vi "sigmoid.vi"(11 "x":dbl) -> (3 "sigmoid(x)":dbl)   [LabVIEW 2019]
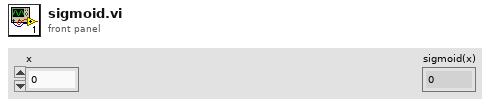
[diagram p1: front panel]
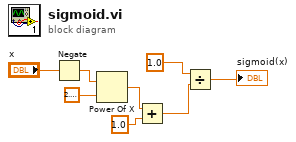
[diagram p0: block diagram]
diagram:
  n1 = Negate(x="x") -> (-x=w3:dbl)
  n2 = Power Of X(1:2.718281828459045, 2:w3) -> (0:w2:dbl)
  n3 = Add(x=w2, y=1.0) -> (x+y=w6:dbl)
  n4 = Divide(x=1.0, y=w6) -> (x/y=→"sigmoid(x)":dbl)
